vi "Initialize RF boards - interlace 3.vi"(2 "error in":errorcluster, 3 "FPGA VI Reference In":T1) -> (0 "error out":errorcluster, 1 "FPGA VI Reference Out":T1)   [LabVIEW 2013]
uses:
  <vilib>/rvi/interface/nirviReadWriteControl/nirviReadWriteControl.xnode
  openfpgaref.8.6.ctl
  NiFpgaLv.dll
  <vilib>/Utility/error.llb/Error Cluster From Error Code.vi
  <vilib>/rvi/errors/niLvFpgaAdjustHostInterfaceError.vi
  FPGA Bitfiles/UHR-FleezersInst_FPGATarget_UHR-Fleezers_Leonardo042018V2.lvbitx
  <vilib>/rvi/errors/niLvFpgaMergeErrorWithErrorCode.vi
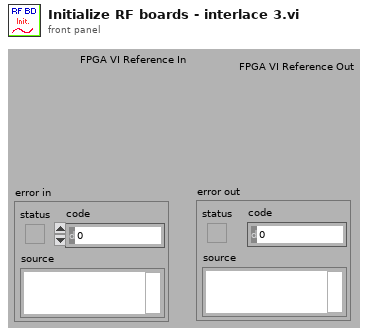
[diagram p1: front panel]
types:
  T1 = typedef "openfpgaref.8.6.ctl" = refnum<k20>
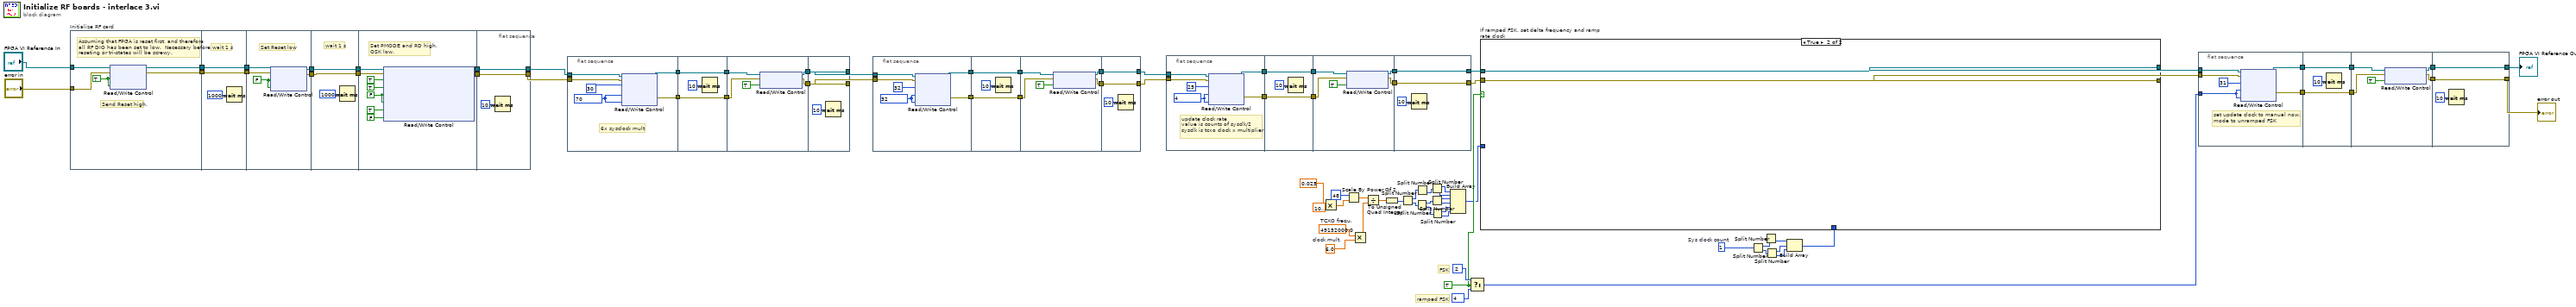
[diagram p0: block diagram]
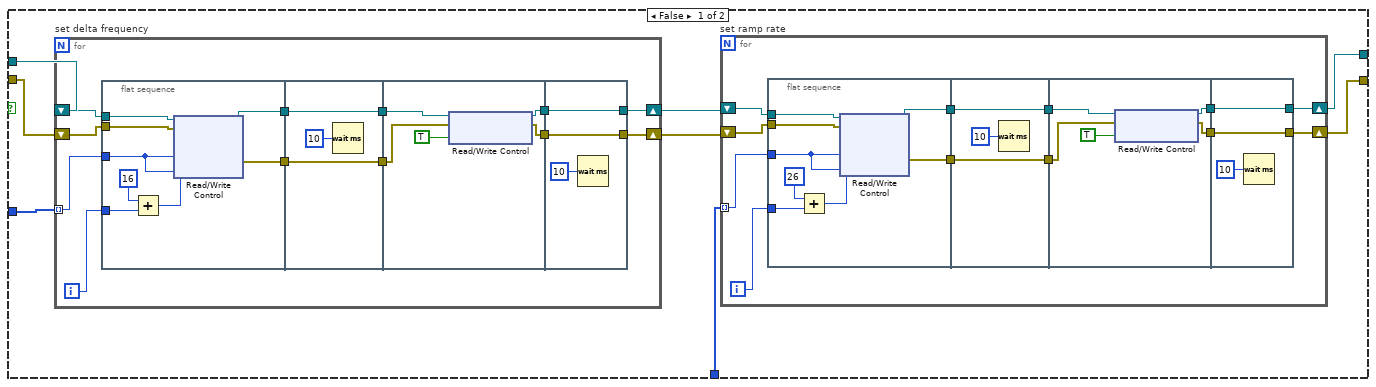
[diagram p2: hidden frame]
diagram:
  w9 = u32 1  # Sys clock count
  w25 = 6.0  # clock mult.
  w26 = 49152000.0  # TCXO frequ.
  w33 = TRUE
  # "ramped FSK"
  # "FSK"
  n1 = flat-sequence "Initialize RF card" {
    tunnel: [w86] -> w81
    tunnel: [w85] -> w80
    tunnel: "error in" -> [w84]
    tunnel: "FPGA VI Reference In" -> [w82]
    tunnel: w81 -> [w88]
    tunnel: w80 -> [w87]
    tunnel: [w88] -> w79
    tunnel: [w87] -> w78
    tunnel: w79 -> [w94]
    tunnel: w78 -> [w93]
    tunnel: [w92] -> w77
    tunnel: [w91] -> w76
    tunnel: w77 -> [w96]
    tunnel: w76 -> [w95]
    tunnel: [w96] -> w75
    tunnel: [w95] -> w74
    tunnel: w75 -> [w106]
    tunnel: w74 -> [w105]
    tunnel: [w102] -> w62
    tunnel: [w101] -> w61
    tunnel: [w108] -> w55
    tunnel: [w109] -> w56
    tunnel: w62 -> [w109]
    tunnel: w61 -> [w108]
    frame #0 {
      w83 = TRUE ("Reset")
      # "Send Reset high."
      # "Assuming that FPGA is reset first, and therefore\nall RF DIO has been set to low.  Necessary before\nreseting or tri-states will be screwy."
      n2 = xnode "Read/Write Control"("FPGA VI Reference In"=w82, "error in"=w84, "Reset Bd 1"=w83, "Reset Bd 2"=w83) -> ("FPGA VI Reference Out"=w86:T1, "error out"=w85:errorcluster)
    }
    frame #1 {
      # "wait 1 s"
      n3 = Wait (ms)(milliseconds to wait=u32 1000) -> ()  [unwired: 1 out]
    }
    frame #2 {
      w90 = FALSE ("Reset")
      # "Set Reset low"
      n4 = xnode "Read/Write Control"("FPGA VI Reference In"=w94, "error in"=w93, "Reset Bd 1"=w90, "Reset Bd 2"=w90) -> ("FPGA VI Reference Out"=w92:T1, "error out"=w91:errorcluster)
    }
    frame #3 {
      # "wait 1 s"
      n5 = Wait (ms)(milliseconds to wait=u32 1000) -> ()  [unwired: 1 out]
    }
    frame #4 {
      w100 = FALSE ("OSK")
      # "Set PMODE and RD high,\nOSK low."
      n6 = xnode "Read/Write Control"("FPGA VI Reference In"=w106, "error in"=w105, "RD"=TRUE, "PMODE"=TRUE, "OSK Bd 1"=w100, "OSK Bd 2"=w100, "Direct RF Box  Communication"=TRUE, "FPGA Controls  RF Box"=FALSE) -> ("FPGA VI Reference Out"=w102:T1, "error out"=w101:errorcluster)
    }
    frame #5 {
      n7 = Wait (ms)(milliseconds to wait=u32 10) -> ()  [unwired: 1 out]
    }
  }
  n8 = flat-sequence {
    tunnel: [w115] -> w73
    tunnel: [w114] -> w72
    tunnel: w56 -> [w113]
    tunnel: w55 -> [w112]
    tunnel: [w117] -> w71
    tunnel: w73 -> [w117]
    tunnel: [w116] -> w70
    tunnel: w72 -> [w116]
    tunnel: w71 -> [w123]
    tunnel: w70 -> [w122]
    tunnel: [w120] -> w60
    tunnel: [w119] -> w59
    tunnel: [w125] -> w64
    tunnel: [w126] -> w65
    tunnel: w60 -> [w126]
    tunnel: w59 -> [w125]
    frame #0 {
      w110 = u8 70 ("Data")
      # "6x sysclock mult"
      n9 = xnode "Read/Write Control"("FPGA VI Reference In"=w113, "error in"=w112, "Address"=u8 30, "Data BD 1"=w110, "Data BD 2"=w110) -> ("FPGA VI Reference Out"=w115:T1, "error out"=w114:errorcluster)
    }
    frame #1 {
      n10 = Wait (ms)(milliseconds to wait=u32 10) -> ()  [unwired: 1 out]
    }
    frame #2 {
      n11 = xnode "Read/Write Control"("FPGA VI Reference In"=w123, "error in"=w122, "Update Data"=TRUE) -> ("FPGA VI Reference Out"=w120:T1, "error out"=w119:errorcluster)
    }
    frame #3 {
      n12 = Wait (ms)(milliseconds to wait=u32 10) -> ()  [unwired: 1 out]
    }
  }
  n13 = flat-sequence {
    tunnel: [w132] -> w69
    tunnel: [w131] -> w68
    tunnel: w65 -> [w130]
    tunnel: w64 -> [w129]
    tunnel: [w134] -> w67
    tunnel: w69 -> [w134]
    tunnel: [w133] -> w66
    tunnel: w68 -> [w133]
    tunnel: w67 -> [w140]
    tunnel: w66 -> [w139]
    tunnel: [w137] -> w58
    tunnel: [w136] -> w57
    tunnel: [w142] -> w47
    tunnel: [w143] -> w48
    tunnel: w58 -> [w143]
    tunnel: w57 -> [w142]
    frame #0 {
      w127 = u8 32 ("Data")
      n14 = xnode "Read/Write Control"("FPGA VI Reference In"=w130, "error in"=w129, "Address"=u8 32, "Data BD 1"=w127, "Data BD 2"=w127) -> ("FPGA VI Reference Out"=w132:T1, "error out"=w131:errorcluster)
    }
    frame #1 {
      n15 = Wait (ms)(milliseconds to wait=u32 10) -> ()  [unwired: 1 out]
    }
    frame #2 {
      n16 = xnode "Read/Write Control"("FPGA VI Reference In"=w140, "error in"=w139, "Update Data"=TRUE) -> ("FPGA VI Reference Out"=w137:T1, "error out"=w136:errorcluster)
    }
    frame #3 {
      n17 = Wait (ms)(milliseconds to wait=u32 10) -> ()  [unwired: 1 out]
    }
  }
  n18 = flat-sequence {
    tunnel: [w149] -> w54
    tunnel: [w148] -> w53
    tunnel: w48 -> [w147]
    tunnel: w47 -> [w146]
    tunnel: [w151] -> w52
    tunnel: w54 -> [w151]
    tunnel: [w150] -> w51
    tunnel: w53 -> [w150]
    tunnel: w52 -> [w157]
    tunnel: w51 -> [w156]
    tunnel: [w154] -> w50
    tunnel: [w153] -> w49
    tunnel: [w159] -> w45
    tunnel: [w160] -> w46
    tunnel: w50 -> [w160]
    tunnel: w49 -> [w159]
    frame #0 {
      w144 = u8 4 ("Data")
      # "update clock rate\nvalue is counts of sysclk/2\nsysclk is tcxo clock x multiplier"
      n19 = xnode "Read/Write Control"("FPGA VI Reference In"=w147, "error in"=w146, "Address"=u8 25, "Data BD 1"=w144, "Data BD 2"=w144) -> ("FPGA VI Reference Out"=w149:T1, "error out"=w148:errorcluster)
    }
    frame #1 {
      n20 = Wait (ms)(milliseconds to wait=u32 10) -> ()  [unwired: 1 out]
    }
    frame #2 {
      n21 = xnode "Read/Write Control"("FPGA VI Reference In"=w157, "error in"=w156, "Update Data"=TRUE) -> ("FPGA VI Reference Out"=w154:T1, "error out"=w153:errorcluster)
    }
    frame #3 {
      n22 = Wait (ms)(milliseconds to wait=u32 10) -> ()  [unwired: 1 out]
    }
  }
  n23 = Multiply(x=0.025 ("Delta Frequency  (MHz)"), y=1000000.0) -> (x*y=w28:dbl)
  n24 = Scale By Power Of 2(n=48, x=w28) -> (x*2^n=w30:dbl)
  n25 = Multiply(x=w26, y=w25) -> (x*y=w23:dbl)
  n26 = Divide(x=w30, y=w23) -> (x/y=w29:dbl)
  n27 = To Unsigned Quad Integer(1:w29) -> (0:w22:u64)
  n28 = Split Number(x=w22) -> (hi(x)=w21:u32, lo(x)=w20:u32)
  n29 = Split Number(x=w20) -> (hi(x)=w18:u16, lo(x)=w19:u16)
  n30 = Split Number(x=w21) -> (lo(x)=w17:u16)  [unwired: 1 out]
  n31 = Split Number(x=w17) -> (hi(x)=w16:u8, lo(x)=w15:u8)
  n32 = Split Number(x=w18) -> (hi(x)=w14:u8, lo(x)=w13:u8)
  n33 = Split Number(x=w19) -> (hi(x)=w12:u8, lo(x)=w11:u8)
  n34 = Build Array(w16, w15, w14, w13, w12, w11) -> (w10:u8[])
  n35 = Select(t=u8 2 ("Data"), s=w33, f=u8 4 ("Data")) -> (s? t:f=w34:u8)
  n36 = Split Number(x=w9) -> (hi(x)=w8:u16, lo(x)=w7:u16)
  n37 = Split Number(x=w8) -> (lo(x)=w6:u8)  [unwired: 1 out]
  n38 = Split Number(x=w7) -> (hi(x)=w5:u8, lo(x)=w4:u8)
  n39 = Build Array(w6, w5, w4) -> (w3:u8[])
  n40 = case "If ramped FSK, set delta frequency and ramp rate clock" shown="True" w33 {
    tunnel: w46 -> [w168 w232]
    tunnel: w45 -> [w167 w231]
    tunnel: [w162 w231] -> w42
    tunnel: [w163 w232] -> w41
    tunnel: w10 -> [w166 _]
    tunnel: w3 -> [w161 _]
    frame False {
      n41 = for "set delta frequency" {
        shift-right: [w202] -> w165
        shift-left: w168 -> [w205]
        shift-right: [w203] -> w164
        shift-left: w167 -> [w204]
        tunnel: w166 -> [w200] mode=indexing
        i -> [w201]
        n42 = flat-sequence {
          tunnel: [w219] -> w211
          tunnel: [w218] -> w210
          tunnel: w205 -> [w217]
          tunnel: w204 -> [w216]
          tunnel: w201 -> [w214]
          tunnel: w200 -> [w212]
          tunnel: [w221] -> w209
          tunnel: w211 -> [w221]
          tunnel: [w220] -> w208
          tunnel: w210 -> [w220]
          tunnel: w209 -> [w227]
          tunnel: w208 -> [w226]
          tunnel: [w224] -> w207
          tunnel: [w223] -> w206
          tunnel: [w230] -> w203
          tunnel: [w228] -> w202
          tunnel: w207 -> [w228]
          tunnel: w206 -> [w230]
          frame #0 {
            n43 = Add(x=u8 16 ("Address"), y=w214) -> (x+y=w213:i32)
            n44 = xnode "Read/Write Control"("FPGA VI Reference In"=w217, "error in"=w216, "Address"=w213, "Data BD 1"=w212, "Data BD 2"=w212) -> ("FPGA VI Reference Out"=w219:T1, "error out"=w218:errorcluster)
          }
          frame #1 {
            n45 = Wait (ms)(milliseconds to wait=u32 10) -> ()  [unwired: 1 out]
          }
          frame #2 {
            n46 = xnode "Read/Write Control"("FPGA VI Reference In"=w227, "error in"=w226, "Update Data"=TRUE) -> ("FPGA VI Reference Out"=w224:T1, "error out"=w223:errorcluster)
          }
          frame #3 {
            n47 = Wait (ms)(milliseconds to wait=u32 10) -> ()  [unwired: 1 out]
          }
        }
      }
      n48 = for "set ramp rate" {
        shift-right: [w171] -> w163
        shift-left: w165 -> [w174]
        shift-right: [w172] -> w162
        shift-left: w164 -> [w173]
        tunnel: w161 -> [w169] mode=indexing
        i -> [w170]
        n49 = flat-sequence {
          tunnel: [w188] -> w180
          tunnel: [w187] -> w179
          tunnel: w174 -> [w186]
          tunnel: w173 -> [w185]
          tunnel: w170 -> [w183]
          tunnel: w169 -> [w181]
          tunnel: [w190] -> w178
          tunnel: w180 -> [w190]
          tunnel: [w189] -> w177
          tunnel: w179 -> [w189]
          tunnel: w178 -> [w196]
          tunnel: w177 -> [w195]
          tunnel: [w193] -> w176
          tunnel: [w192] -> w175
          tunnel: [w199] -> w172
          tunnel: [w197] -> w171
          tunnel: w176 -> [w197]
          tunnel: w175 -> [w199]
          frame #0 {
            n50 = Add(x=u8 26 ("Address"), y=w183) -> (x+y=w182:i32)
            n51 = xnode "Read/Write Control"("FPGA VI Reference In"=w186, "error in"=w185, "Address"=w182, "Data BD 1"=w181, "Data BD 2"=w181) -> ("FPGA VI Reference Out"=w188:T1, "error out"=w187:errorcluster)
          }
          frame #1 {
            n52 = Wait (ms)(milliseconds to wait=u32 10) -> ()  [unwired: 1 out]
          }
          frame #2 {
            n53 = xnode "Read/Write Control"("FPGA VI Reference In"=w196, "error in"=w195, "Update Data"=TRUE) -> ("FPGA VI Reference Out"=w193:T1, "error out"=w192:errorcluster)
          }
          frame #3 {
            n54 = Wait (ms)(milliseconds to wait=u32 10) -> ()  [unwired: 1 out]
          }
        }
      }
    }
    frame True {
    }
  }
  n55 = flat-sequence {
    tunnel: [w238] -> w40
    tunnel: [w237] -> w39
    tunnel: w41 -> [w236]
    tunnel: w42 -> [w235]
    tunnel: w34 -> [w233]
    tunnel: [w240] -> w38
    tunnel: w40 -> [w240]
    tunnel: [w239] -> w37
    tunnel: w39 -> [w239]
    tunnel: w38 -> [w246]
    tunnel: w37 -> [w245]
    tunnel: [w243] -> w36
    tunnel: [w242] -> w35
    tunnel: [w248] -> w32
    tunnel: [w249] -> w2
    tunnel: w36 -> [w249]
    tunnel: w35 -> [w248]
    frame #0 {
      # "set update clock to manual now,\nmode to unramped FSK"
      n56 = xnode "Read/Write Control"("FPGA VI Reference In"=w236, "error in"=w235, "Address"=u8 31, "Data BD 1"=w233, "Data BD 2"=w233) -> ("FPGA VI Reference Out"=w238:T1, "error out"=w237:errorcluster)
    }
    frame #1 {
      n57 = Wait (ms)(milliseconds to wait=u32 10) -> ()  [unwired: 1 out]
    }
    frame #2 {
      n58 = xnode "Read/Write Control"("FPGA VI Reference In"=w246, "error in"=w245, "Update Data"=TRUE) -> ("FPGA VI Reference Out"=w243:T1, "error out"=w242:errorcluster)
    }
    frame #3 {
      n59 = Wait (ms)(milliseconds to wait=u32 10) -> ()  [unwired: 1 out]
    }
  }
  "error out" <- w32
  "FPGA VI Reference Out" <- w2
